vi "Initialize.vi"(0 "Universal Power Meter in":refnum<class "Universal Power Meter.lvclass">, 7 "Reset (T: Reset)":bool=TRUE, 9 "ID Query (T: Check)":bool=TRUE, 11 "error in (no error)":errorcluster) -> (4 "Universal Power Meter out":refnum<class "Universal Power Meter.lvclass">, 6 "VISA resource name":refnum<visa-resource-name>, 15 "error out":errorcluster)   [LabVIEW 2014, in "Universal Power Meter.lvlib" / "Universal Power Meter.lvclass"]
uses:
  Universal Power Meter.lvclass
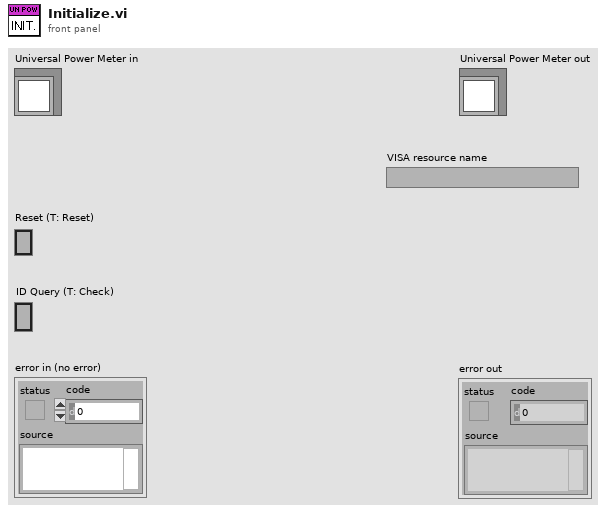
[diagram p1: front panel]
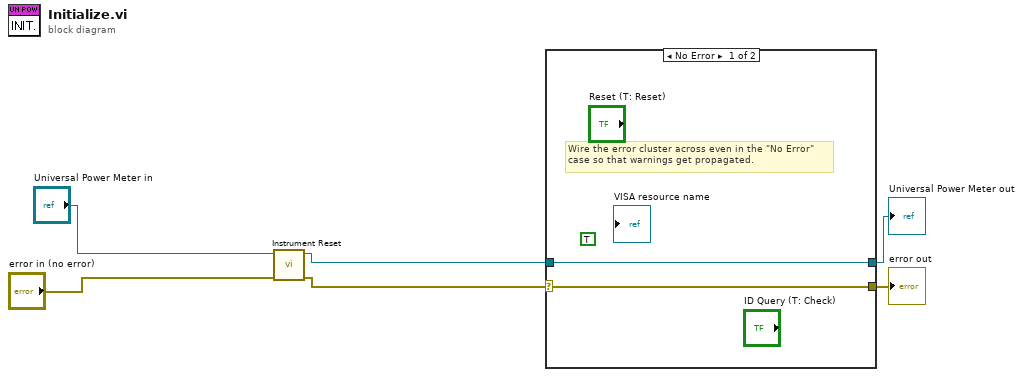
[diagram p0: block diagram]
diagram:
  n1 = call-dynamic "Instrument Reset.vi"("error in (no error)"="error in (no error)", "Universal Power Meter in"="Universal Power Meter in") -> ("error out"=w2:errorcluster, "Universal Power Meter out"=w3:refnum<class "Universal Power Meter.lvclass">)  [unwired: 8 in]
  n2 = case shown="No Error" w2 {
    selector: w2 -> [w7 w10]
    tunnel: [w7 w10] -> w6
    tunnel: [w8 w9] -> w1
    tunnel: w3 -> [w8 w9]
    frame No Error {
      (unwired) TRUE ("On/Off")
      # "Wire the error cluster across even in the \"No Error\"\ncase so that warnings get propagated."
    }
    frame Error {
    }
  }
  "error out" <- w6
  "Universal Power Meter out" <- w1
